vi "BuildLinkSettings.vi"(0 "Twist":T1, 2 "Pose":T2, 3 "link to move":string="boxes::link1") -> (4 "msg out":string)   [LabVIEW 2012]
uses:
  <userlib>/rosforlv/ROS/MessageBuilding/std_msgs/subs/stringScalar.vi
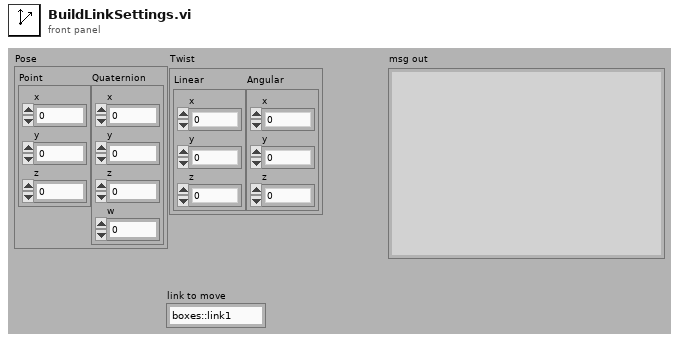
[diagram p1: front panel]
types:
  T1 = cluster{"Linear":cluster{"x":dbl, "y":dbl, "z":dbl}, "Angular":cluster{"x":dbl, "y":dbl, "z":dbl}}
  T2 = cluster{"Point":cluster{"x":dbl, "y":dbl, "z":dbl}, "Quaternion":cluster{"x":dbl, "y":dbl, "z":dbl, "w":dbl}}
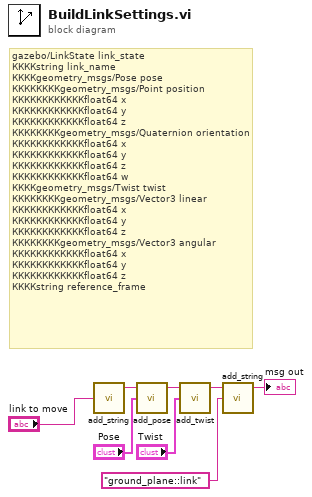
[diagram p0: block diagram]
diagram:
  # "gazebo/LinkState link_state\nККККstring link_name\nККККgeometry_msgs/Pose pose\nККККККККgeometry_msgs/Point position\nККККККККККККfloat64 x\nККККККККККККfloat64 y\nККККККККККККfloat64 z\nККККККККgeometry_msgs/Quaternion orientation\nККККККККККККfloat64 x\nККККККККККККfloat64 y\nККККККККККККfloat64 z\nККККККККККККfloat64 w\nККККgeometry_msgs/Twist twist\nККККККККgeometry_msgs/Vector3 linear\nККККККККККККfloat64 x\nККККККККККККfloat64 y\nККККККККККККfloat64 z\nККККККККgeometry_msgs/Vector3 angular\nККККККККККККfloat64 x\nККККККККККККfloat64 y\nККККККККККККfloat64 z\nККККstring reference_frame"
  n1 = call-poly <userlib>:"add_string.vi"("String"="link to move") -> ("msg out"=w6:string)  [unwired: 4 in]
  n2 = call <userlib>:"add_pose.vi"("Pose"="Pose", "msg in"=w6) -> ("msg out"=w7:string)  [unwired: 3 in]
  n3 = call <userlib>:"add_twist.vi"("Twist"="Twist", "msg in"=w7) -> ("msg out"=w4:string)  [unwired: 3 in]
  n4 = call-poly <userlib>:"add_string.vi"("String"="ground_plane::link", "msg in"=w4) -> ("msg out"=→"msg out":string)  [unwired: 3 in]
